vi "Delete Session Refnum.vi"(8 "error in (no error)":errorcluster, 11 "session":T1) -> (0 "error out":errorcluster, 3 "LIBSSH2_SESSION*":u64)   [LabVIEW 2017, in "libssh2.lvlib"]
uses:
  libssh2.lvlib
  Session Refnum.ctl
  Session Refnum Data.ctl
  libssh2_session_abstract.ctl
  lvssh2_session_callback_events.ctl
  lvssh2_session_callback_send_function_input_args_32.ctl
  lvssh2_session_callback_receive_function_input_args_32.ctl
  lvssh2_userauth_keyboard_interactive_response_function_input_args_32.ctl
  lvssh2_session_callback_send_function_input_args_64.ctl
  lvssh2_session_callback_receive_function_input_args_64.ctl
  lvssh2_userauth_keyboard_interactive_response_function_input_args_64.ctl
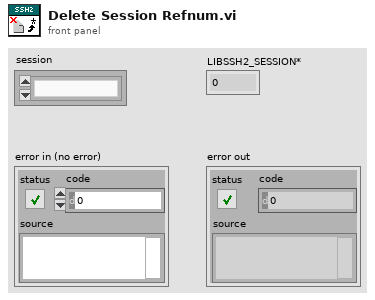
[diagram p1: front panel]
types:
  T1 = typedef "libssh2.lvlib/Session Refnum.ctl" = refnum<k1>
  T2 = typedef "libssh2.lvlib/Session Refnum Data.ctl" = cluster{"LIBSSH2_SESSION*":u64, "abstract":T3, "events":T4, "semaphore":T5}
  T3 = typedef "libssh2.lvlib/libssh2_session_abstract.ctl" = cluster{"send":refnum<vi>, "receive":refnum<vi>, "keyboard-interactive response":refnum<vi>}
  T4 = typedef "libssh2.lvlib/lvssh2_session_callback_events.ctl" = cluster{"32-bit":cluster{"send":refnum<user-event>, "recv":refnum<user-event>, "kbdint_response":refnum<user-event>}, "64-bit":cluster{"send":refnum<user-event>, "recv":refnum<user-event>, "kbdint_response":refnum<user-event>}, "stop":cluster{"send":refnum<user-event>, "recv":refnum<user-event>, "kbdint_response":refnum<user-event>}}
  T5 = typedef "Semaphore RefNum" = refnum<k1>
  T6 = cluster{"send":refnum<user-event>, "recv":refnum<user-event>, "kbdint_response":refnum<user-event>}
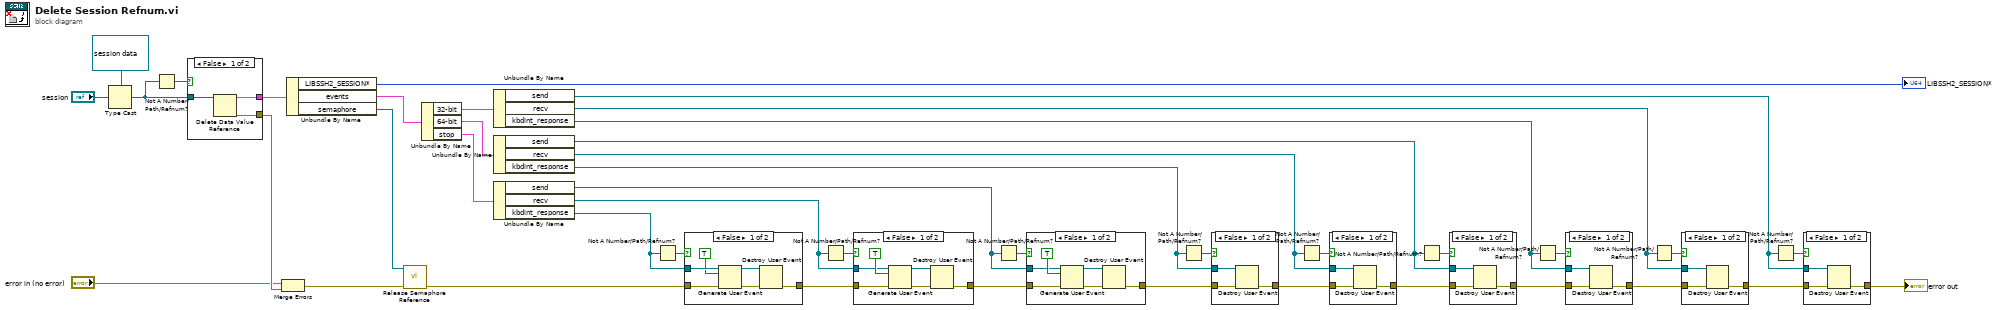
[diagram p0: block diagram]
diagram:
  n1 = Type Cast(type=refnum<data-value> refnum ("data value reference"), x="session") -> (*(type *) &x=w39:refnum<data-value>)
  n2 = Not A Number/Path/Refnum?(number/path/refnum=w39) -> (NaN/Path/Refnum?=w38:bool)
  n3 = case shown="False" w38 {
    tunnel: [w45 _] -> w41
    tunnel: [w44 _] -> w40
    tunnel: w39 -> [w43 _]
    frame False {
      n4 = Delete Data Value Reference(data value reference=w43) -> (data value=w45:T2, error out=w44:errorcluster)  [unwired: 1 in]
    }
    frame True {
    }
  }
  n5 = Merge Errors("error in (no error)", w40) -> (w13:errorcluster)
  n6 = Unbundle By Name(w41) -> ("LIBSSH2_SESSION*"=→"LIBSSH2_SESSION*":u64, "events"=w33:T4, "semaphore"=w12:T5)
  n7 = call <vilib>:"Release Semaphore Reference.vi"("error in (no error)"=w13, "semaphore"=w12) -> ("error out"=w1:errorcluster)  [unwired: 8 in, 1 out]
  n8 = Unbundle By Name(w33) -> ("32-bit"=w25:T6, "64-bit"=w30:T6, "stop"=w2:T6)
  n9 = Unbundle By Name(w25) -> ("send"=w24:refnum<user-event>, "recv"=w21:refnum<user-event>, "kbdint_response"=w15:refnum<user-event>)
  n10 = Unbundle By Name(w30) -> ("send"=w29:refnum<user-event>, "recv"=w26:refnum<user-event>, "kbdint_response"=w19:refnum<user-event>)
  n11 = Unbundle By Name(w2) -> ("send"=w5:refnum<user-event>, "recv"=w8:refnum<user-event>, "kbdint_response"=w10:refnum<user-event>)
  n12 = Not A Number/Path/Refnum?(number/path/refnum=w10) -> (NaN/Path/Refnum?=w9:bool)
  n13 = case shown="False" w9 {
    tunnel: [w51 w52] -> w11
    tunnel: w10 -> [w48 _]
    tunnel: w1 -> [w50 w52]
    frame False {
      n14 = Generate User Event(user event=w48, event data cluster=TRUE ("event data"), error in=w50) -> (user event out=w47:refnum<user-event>, error out=w49:errorcluster)  [unwired: 1 in]
      n15 = Destroy User Event(user event=w47, error in=w49) -> (error out=w51:errorcluster)
    }
    frame True {
    }
  }
  n16 = Not A Number/Path/Refnum?(number/path/refnum=w8) -> (NaN/Path/Refnum?=w6:bool)
  n17 = case shown="False" w6 {
    tunnel: w11 -> [w55 w59]
    tunnel: [w58 w59] -> w7
    tunnel: w8 -> [w56 _]
    frame False {
      n18 = Generate User Event(user event=w56, event data cluster=TRUE ("event data"), error in=w55) -> (user event out=w53:refnum<user-event>, error out=w54:errorcluster)  [unwired: 1 in]
      n19 = Destroy User Event(user event=w53, error in=w54) -> (error out=w58:errorcluster)
    }
    frame True {
    }
  }
  n20 = Not A Number/Path/Refnum?(number/path/refnum=w5) -> (NaN/Path/Refnum?=w4:bool)
  n21 = case shown="False" w4 {
    tunnel: w7 -> [w63 w66]
    tunnel: [w65 w66] -> w3
    tunnel: w5 -> [w62 _]
    frame False {
      n22 = Generate User Event(user event=w62, event data cluster=TRUE ("event data"), error in=w63) -> (user event out=w61:refnum<user-event>, error out=w60:errorcluster)  [unwired: 1 in]
      n23 = Destroy User Event(user event=w61, error in=w60) -> (error out=w65:errorcluster)
    }
    frame True {
    }
  }
  n24 = Not A Number/Path/Refnum?(number/path/refnum=w19) -> (NaN/Path/Refnum?=w20:bool)
  n25 = case shown="False" w20 {
    tunnel: w3 -> [w69 w70]
    tunnel: [w68 w70] -> w14
    tunnel: w19 -> [w67 _]
    frame False {
      n26 = Destroy User Event(user event=w67, error in=w69) -> (error out=w68:errorcluster)
    }
    frame True {
    }
  }
  n27 = Not A Number/Path/Refnum?(number/path/refnum=w26) -> (NaN/Path/Refnum?=w28:bool)
  n28 = case shown="False" w28 {
    tunnel: w14 -> [w73 w74]
    tunnel: [w72 w74] -> w27
    tunnel: w26 -> [w71 _]
    frame False {
      n29 = Destroy User Event(user event=w71, error in=w73) -> (error out=w72:errorcluster)
    }
    frame True {
    }
  }
  n30 = Not A Number/Path/Refnum?(number/path/refnum=w29) -> (NaN/Path/Refnum?=w32:bool)
  n31 = case shown="False" w32 {
    tunnel: w27 -> [w77 w78]
    tunnel: [w76 w78] -> w17
    tunnel: w29 -> [w75 _]
    frame False {
      n32 = Destroy User Event(user event=w75, error in=w77) -> (error out=w76:errorcluster)
    }
    frame True {
    }
  }
  n33 = Not A Number/Path/Refnum?(number/path/refnum=w15) -> (NaN/Path/Refnum?=w18:bool)
  n34 = case shown="False" w18 {
    tunnel: w17 -> [w81 w82]
    tunnel: [w80 w82] -> w16
    tunnel: w15 -> [w79 _]
    frame False {
      n35 = Destroy User Event(user event=w79, error in=w81) -> (error out=w80:errorcluster)
    }
    frame True {
    }
  }
  n36 = Not A Number/Path/Refnum?(number/path/refnum=w21) -> (NaN/Path/Refnum?=w23:bool)
  n37 = case shown="False" w23 {
    tunnel: w16 -> [w85 w86]
    tunnel: [w84 w86] -> w22
    tunnel: w21 -> [w83 _]
    frame False {
      n38 = Destroy User Event(user event=w83, error in=w85) -> (error out=w84:errorcluster)
    }
    frame True {
    }
  }
  n39 = Not A Number/Path/Refnum?(number/path/refnum=w24) -> (NaN/Path/Refnum?=w31:bool)
  n40 = case shown="False" w31 {
    tunnel: w22 -> [w89 w90]
    tunnel: [w88 w90] -> w34
    tunnel: w24 -> [w87 _]
    frame False {
      n41 = Destroy User Event(user event=w87, error in=w89) -> (error out=w88:errorcluster)
    }
    frame True {
    }
  }
  "error out" <- w34
